vi "Set_Tunnel_Speed_Multi.vi"(3 "Simulate/Run":T3, 5 "Traverse line":T4 {"Carrier_2 Q (l/min)" format="%#.2f"; "Row Duration (mins)" format="%#.1f"; "Row No" min=0; "Trace Gas Concentration (%)" min=0.0 format="%#_4f"; "Carrier_1 Q (l/min)" format="%#.4f"; "Start X" format="%#.2f"; "Start Y" format="%#.2f"; "Start Z" format="%#.2f"; "End X" format="%#.2f"; "End Y" format="%#.2f"; "End Z" format="%#.2f"; "Tunnel Speed" format="%#.2f"; "Averaging time (mins)" min=0.0 format="%#.2f"}) -> (0 "Status Cluster":T1, 2 "Tunnel speed set?":bool)   [LabVIEW 2020]
uses:
  Traverse_cluster.ctl
  Spacing.ctl
  Controls/Multi_run_mode.ctl
  Controls/User_Specific_mode.ctl
  Status_Cluster.ctl
  Multi_Run_Status.ctl
  ADAM Client/Sub VIs/ADAM Controls/Tunnel_speed_mode.ctl
  Globals/Preference_global.vi
  Globals/Extra_Commands_Global.vi
panel:
  # "X           Y          Z"
  # "Start"
  # "End"
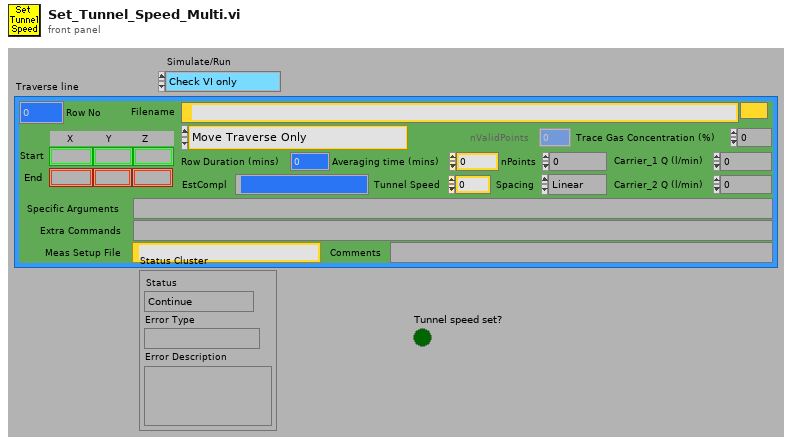
[diagram p1: front panel]
types:
  T1 = typedef "Status_Cluster.ctl" = cluster{"Status":T2, "Error Type":string, "Error Description":string}
  T2 = typedef "Multi_Run_Status.ctl" = enum16{"Continue", "Continue with Error", "Jump to Next Point", "Jump to Next Row", "Jump To Fall Back", "Terminate Run"}
  T3 = typedef "User_Specific_mode.ctl" = enum16{"Check VI only", "Run VI"}
  T4 = typedef "Traverse_cluster.ctl" = cluster{"Start X":sgl, "Start Y":sgl, "Start Z":sgl, "End X":sgl, "End Y":sgl, "End Z":sgl, "nPoints":i32, "Spacing":T5, "Filename":path, "Tunnel Speed":dbl, "Averaging time (mins)":dbl, "Extra Commands":string, "Carrier_1 Q (l/min)":dbl, "Carrier_2 Q (l/min)":dbl, "Trace Gas Concentration (%)":dbl, "Specific Arguments":string, "Comments":string, "Row No":i32, "Row Type Selector":T6, "EstCompl":string, "Row Duration (mins)":dbl, "nValidPoints":i32, "Meas Setup File":string}
  T5 = typedef "Spacing.ctl" = enum16{"Linear", "Log", "Gauss", "Specified", "N/A"}
  T6 = typedef "Multi_run_mode.ctl" = enum16{"Move Traverse Only", "Set Tunnel Speed Only", "Set Source Only", "Set Measurement Conditions", "Single Measurement", "Vertical Profile", "Lateral Profile", "Longitudinal Profile", "Multi-Axis Profile", "Explore Volume", "Auto Calibrate", "Meas Fast FID Bkgnd", "Check Beam Power", "Scanning Valve Measurement", "Run VI Named:", "Set ADAM Ch", "Wait (minutes)", "Send Message", "Synchronize With:", "Fall Back to this Row", "Turn Off Row Repeating", "Traverse 3D Volume", "Blank Row", "Jump to Fall Back Row"}
  T7 = typedef "Tunnel_speed_mode.ctl" = enum16{"Set Speed", "Set Speed then wait", "Is tunnel speed allowable?"}
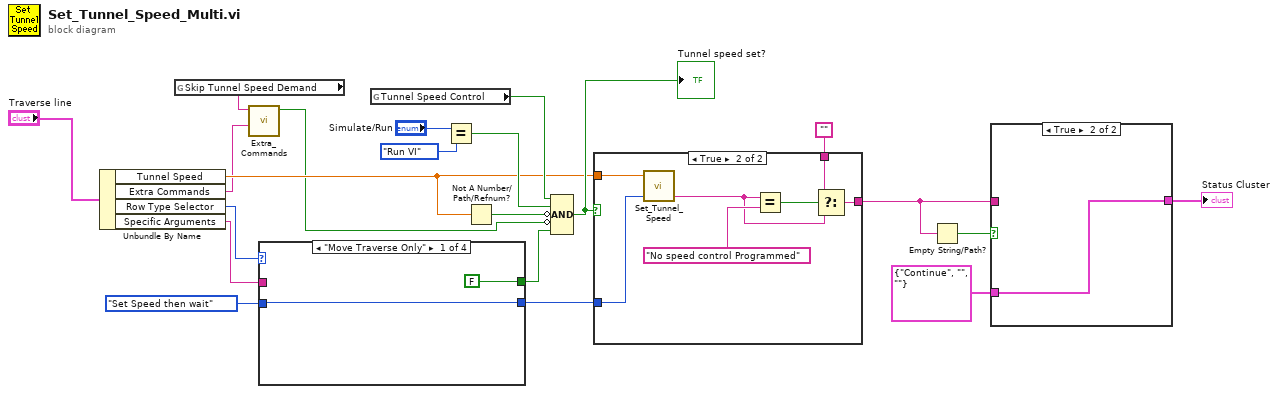
[diagram p0: block diagram]
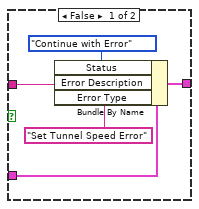
[diagram p2: hidden frame]
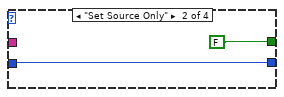
[diagram p3: hidden frame]
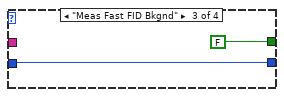
[diagram p4: hidden frame]
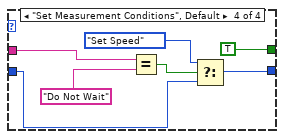
[diagram p5: hidden frame]
diagram:
  n1 = Unbundle By Name("Traverse line") -> ("Tunnel Speed"=w6:dbl, "Extra Commands"=w2:string, "Row Type Selector"=w17:T6, "Specific Arguments"=w4:string)
  n2 = global read "Extra_Commands_Global.vi" "Skip Tunnel Speed Demand"() -> (w3:string)
  n3 = call "Extra_Commands.vi"("String to Search"=w2, "Command"=w3) -> ("Command Found"=w1:bool)  [unwired: 1 in, 4 out]
  n4 = case shown="\"Move Traverse Only\"" w17 {
    tunnel: [FALSE FALSE FALSE TRUE] -> w9
    tunnel: [w22 w24 w26 w28] -> w15
    tunnel: Tunnel_speed_mode."Set Speed then wait" ("Mode") -> [w22 w24 w26 w29]
    tunnel: w4 -> [_ _ _ w33]
    frame "Move Traverse Only" {
    }
    frame "Set Source Only" {
    }
    frame "Meas Fast FID Bkgnd" {
    }
    frame "Set Measurement Conditions", Default {
      n5 = Equal?(x=w33, y="Do Not Wait") -> (x = y?=w31:bool)
      n6 = Select(t=Tunnel_speed_mode."Set Speed" ("Mode"), s=w31, f=w29) -> (s? t:f=w28:T7)
    }
  }
  n7 = global read "Preference_global.vi" "Tunnel Speed Control"() -> (w7:bool)
  n8 = Equal?(x="Simulate/Run", y=User_Specific_mode."Run VI" ("Simulate/Run")) -> (x = y?=w19:bool)
  n9 = Not A Number/Path/Refnum?(number/path/refnum=w6) -> (NaN/Path/Refnum?=w5:bool)
  n10 = Compound Arithmetic op=AND(w7, w19, invert w5, invert w1, w9) -> (w20:bool)
  "Tunnel speed set?" <- w20
  n11 = case shown="True" w20 {
    tunnel: w6 -> [_ w36]
    tunnel: w15 -> [_ w42]
    tunnel: [w35 w37] -> w10
    tunnel: "" -> [w35 w39]
    frame False {
    }
    frame True {
      n12 = call "Set_Tunnel_Speed.vi"("Mode"=w42, "Tunnel Velocity m/s"=w36) -> ("Error String"=w38:string)  [unwired: 1 in, 2 out]
      n13 = Equal?(x=w38, y="No speed control Programmed" ("Error String")) -> (x = y?=w40:bool)
      n14 = Select(t=w39, s=w40, f=w38) -> (s? t:f=w37:string)
    }
  }
  n15 = Empty String/Path?(string/path=w10) -> (empty?=w12:bool)
  n16 = case shown="True" w12 {
    tunnel: T1 {"Status"=enum."Continue", "Error Type"="", "Error Description"=""} ("Status Cluster") -> [w47 w48]
    tunnel: [w46 w48] -> w11
    tunnel: w10 -> [w44 _]
    frame False {
      n17 = Bundle By Name(cluster=w47, "Status"=Multi_Run_Status."Continue with Error", "Error Description"=w44, "Error Type"="Set Tunnel Speed Error" ("Bundle Element")) -> (w46:T1)
    }
    frame True {
    }
  }
  "Status Cluster" <- w11
